vi "DSCProgIOCloop.vi"() -> ()   [LabVIEW 2011]
uses:
  <vilib>/variable/tagger/epicsserver/API/internal/List PVs (By Ref).vi
  <vilib>/variable/tagger/epicsserver/API/internal/Undeploy EPICS Server (By Ref).vi
  <vilib>/variable/tagger/epicsserver/API/internal/EPICSServerClass/EPICSServer.lvclass
  <vilib>/variable/tagger/epicsserver/API/NI_EPICS_Server.lvlib
  <vilib>/lvdsc/NI_DSC.lvlib
panel:
  in  "data in":dbl
  out "data out 2":dbl
  out "data out":dbl
  out "PVs":string[](array[string])
  out "error out":errorcluster
  in  "stop":bool
  out "EPICS Server URL out":string
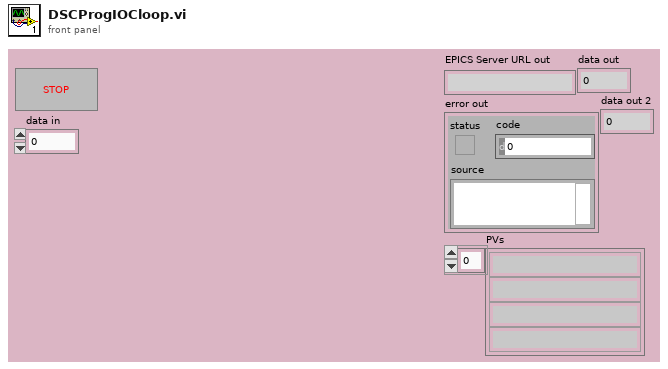
[diagram p1: front panel]
types:
  T1 = enum32{"u32BitField", "bool", "double", "string", "int8", "uint8", "int16", "uint16", "int32", "uint32", "int64", "uint64", "single", "double waveform", "int16 waveform", "array of boolean", "array of int8", "array of uint8", "array of int16", "array of uint16", "array of int32", "array of uint32", "array of int64", "array of uint64", "array of single", "array of double", "array of double waveform", "array of int16 waveform", "array of string", "variant", "timestamp", "fixed point", "custom"}
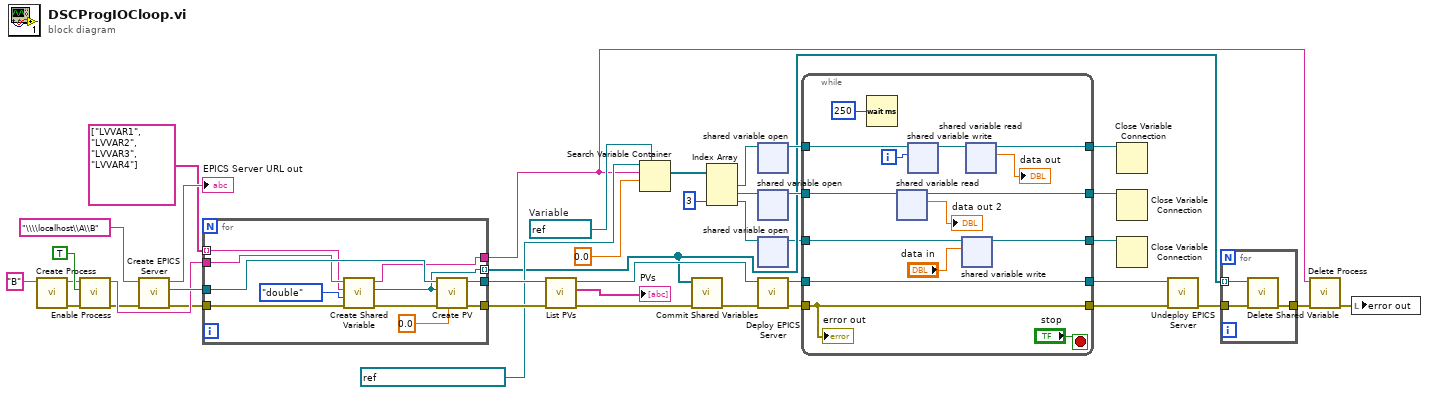
[diagram p0: block diagram]
diagram:
  w25 = refnum<k21> refnum  # Variable
  n1 = call <vilib>:"Create Process.vi"("process name"="B") -> ("error out"=w19:errorcluster, "process name out"=w15:string)  [unwired: 9 in]
  n2 = call <vilib>:"Enable Process.vi"("error in (no error)"=w19, "run?"=TRUE, "process name"=w15) -> ("error out"=w8:errorcluster, "process name out"=w14:string)  [unwired: 7 in]
  n3 = call <vilib>:"Create EPICS Server.vi"("error in (no error)"=w8, "EPICS Server URL in"="\\\\localhost\\A\\B") -> ("error out"=w7:errorcluster, "EPICS Server ref"=w40:refnum<data-value>, "EPICS Server URL out"=→"EPICS Server URL out":string)  [unwired: 7 in]
  n4 = for {
    tunnel: w40 -> [w51]
    tunnel: [w49] -> w35
    tunnel: [w48] -> w34
    tunnel: [w46] -> w16
    tunnel: w14 -> [w45]
    tunnel: [w44] -> w6 mode=indexing
    tunnel: string[] ["LVVAR1", "LVVAR2", "LVVAR3", "LVVAR4"] -> [w43] mode=indexing
    tunnel: w7 -> [w42]
    n5 = call <vilib>:"Create Shared Variable.vi"("error in (no error)"=w42, "data type"=T1."double", "shared variable name"=w43, "process name"=w45) -> ("error out"=w41:errorcluster, "shared variable"=w44:refnum<k21>, "process name out"=w46:string)  [unwired: 5 in]
    n6 = call <vilib>:"Create PV.vi"("data type"=0.0, "error in (no error)"=w41, "variable path"=w44, "EPICS Server ref in"=w51) -> ("error out"=w48:errorcluster, "EPICS Server ref out"=w49:refnum<data-value>)  [unwired: 6 in]
  }
  n7 = call-poly <vilib>:"List PVs.vi"("error in (no error)"=w34, "EPICS Server ref in"=w35) -> ("error out"=w13:errorcluster, "PVs"=→"PVs":string[], "EPICS Server ref out"=w32:refnum<data-value>)  [unwired: 7 in]
  n8 = Search Variable Container(7:w25, 9:0.0, 10:w16, 11:refnum<k21> "ni.var.psp://localhost/" ("container refnum in")) -> (2:w29:refnum<k21>[])  [unwired: 2 in, 2 out]
  n9 = call <vilib>:"Commit Shared Variables.vi"("error in (no error)"=w13, "shared variables"=w6) -> ("error out"=w23:errorcluster)  [unwired: 8 in, 1 out]
  n10 = Index Array(array=w29, index #3=3 ("index")) -> (element #1=w24:refnum<k21>, element #2=w12:refnum<k21>, element #3=w3:refnum<k21>)  [unwired: 2 in]
  n11 = shared-variable-open(w24) -> (w27:refnum<k21>)  [unwired: 2 in, 1 out]
  n12 = shared-variable-open(w12) -> (w11:refnum<k21>)  [unwired: 2 in, 1 out]
  n13 = shared-variable-open(w3) -> (w2:refnum<k21>)  [unwired: 2 in, 1 out]
  n14 = call <vilib>:"Deploy EPICS Server.vi"("error in (no error)"=w23, "EPICS Server ref in"=w32) -> ("error out"=w31:errorcluster, "EPICS Server ref out"=w38:refnum<data-value>)  [unwired: 8 in]
  n15 = while {
    tunnel: w38 -> [w65]
    tunnel: [w65] -> w37
    tunnel: [w64] -> w36
    tunnel: w31 -> [w64]
    tunnel: w27 -> [w62]
    tunnel: [w59] -> w26
    tunnel: w11 -> [w57]
    tunnel: [w56] -> w10
    tunnel: w2 -> [w54]
    tunnel: [w52] -> w1
    i -> [w63]
    stop <- "stop" stop-if-true
    n16 = Wait (ms)(milliseconds to wait=u32 250) -> ()  [unwired: 1 out]
    n17 = shared-variable-read(w57) -> (w56:refnum<k21>, →"data out 2":dbl)  [unwired: 1 in, 2 out]
    n18 = shared-variable-write(w62, w63) -> (w61:refnum<k21>)  [unwired: 1 in, 1 out]
    n19 = shared-variable-write(w54, "data in") -> (w52:refnum<k21>)  [unwired: 1 in, 1 out]
    n20 = shared-variable-read(w61) -> (w59:refnum<k21>, →"data out":dbl)  [unwired: 1 in, 2 out]
    "error out" <- w64
  }
  n21 = Close Variable Connection(11:w26) -> ()  [unwired: 1 in, 1 out]
  n22 = Close Variable Connection(11:w10) -> ()  [unwired: 1 in, 1 out]
  n23 = Close Variable Connection(11:w1) -> ()  [unwired: 1 in, 1 out]
  n24 = call-poly <vilib>:"Undeploy EPICS Server.vi"("error in (no error)"=w36, "EPICS Server ref"=w37) -> ("error out"=w30:errorcluster)  [unwired: 9 in]
  n25 = for {
    tunnel: w30 -> [w69]
    tunnel: [w68] -> w22
    tunnel: w6 -> [w67] mode=indexing
    n26 = call <vilib>:"Delete Shared Variable.vi"("error in (no error)"=w69, "shared variable"=w67) -> ("error out"=w68:errorcluster)  [unwired: 9 in]
  }
  n27 = call <vilib>:"Delete Process.vi"("error in (no error)"=w22, "process name"=w16) -> ("error out"=w5:errorcluster)  [unwired: 9 in]
  n28 = local write "error out"(w5) -> ()
